vi "IsItemDecendant.vi"(8 "error in (no error)":errorcluster, 9 "Item to compare":refnum<class "ILabVIEWItem.lvclass">, 10 "Parent check?":bool, 11 "ILabVIEWItem in":refnum<class "ILabVIEWItem.lvclass">) -> (0 "error out":errorcluster, 2 "Is a decendant?":bool, 3 "ILabVIEWItem out":refnum<class "ILabVIEWItem.lvclass">)   [LabVIEW 2020, in "LabVIEWObjectInterfaces.lvlib" / "ILabVIEWItem.lvclass"]
uses:
  ILabVIEWItem.lvclass
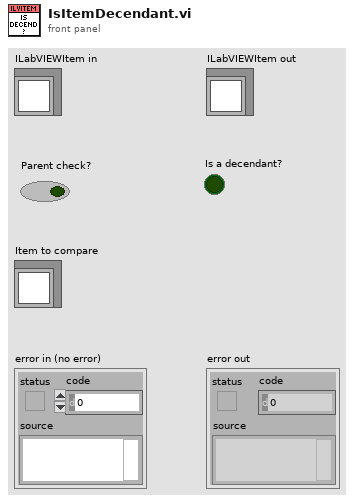
[diagram p1: front panel]
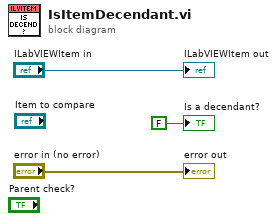
[diagram p0: block diagram]
diagram:
  "error out" <- "error in (no error)"
  "ILabVIEWItem out" <- "ILabVIEWItem in"
  "Is a decendant?" <- FALSE ("Is a decendant?")
